vi "what_do_you_want_checkver.vi"() -> (0 "Next state":T1(ring)=enum."end", 1 "Leave":bool=TRUE)   [LabVIEW 2014]
panel:
  in  "Cluster":cluster{"OK Button 2":bool, "stop":bool}
  # "You have pressed the cancel buttom.\nWhat do you want to do now?\n1.Choose another movie.\n2.Leave the movie booking system"
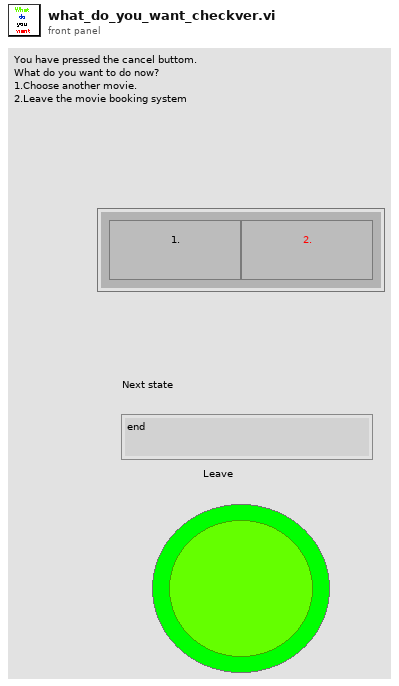
[diagram p1: front panel]
types:
  T1 = enum16{"initial", "start", "member?", "register?", "member login", "member register", "choose movie", "how many seat?", "check", "end"}
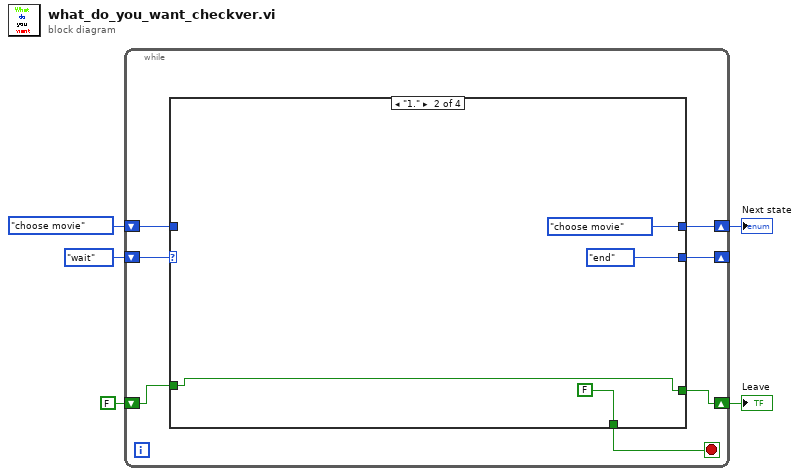
[diagram p0: block diagram]
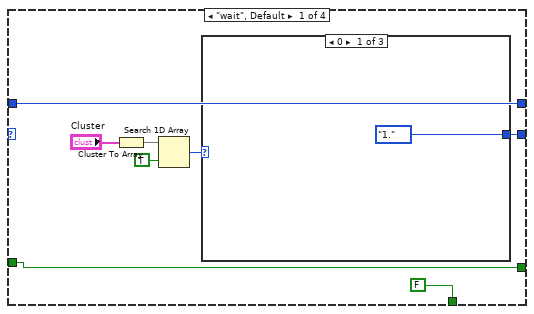
[diagram p2: hidden frame]
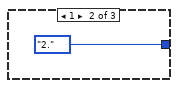
[diagram p3: hidden frame]
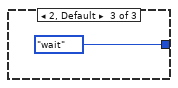
[diagram p4: hidden frame]
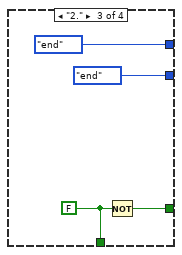
[diagram p5: hidden frame]
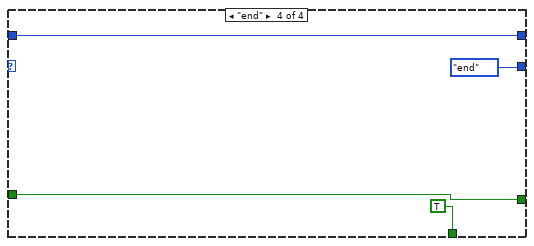
[diagram p6: hidden frame]
diagram:
  n1 = while {
    shift-right: [w11] -> _
    shift-left: enum16{"wait", "1.", "2.", "3.", "end"}."wait" -> [w12]
    shift-right: [w9] -> w3
    shift-left: T1."choose movie" -> [w10]
    shift-right: [w7] -> w1
    shift-left: FALSE -> [w6]
    stop <- w8 stop-if-true
    n2 = case shown="\"1.\"" w12 {
      tunnel: [w16 enum16{"wait", "1.", "2.", "3.", "end"}."end" enum16{"wait", "1.", "2.", "3.", "end"}."end" enum16{"wait", "1.", "2.", "3.", "end"}."end"] -> w11
      tunnel: [w15 T1."choose movie" T1."end" w34] -> w9
      tunnel: w10 -> [w15 _ _ w34]
      tunnel: [FALSE FALSE w29 TRUE] -> w8
      tunnel: [w13 w24 w28 w32] -> w7
      tunnel: w6 -> [w13 w24 _ w32]
      frame "wait", Default {
        n3 = Cluster To Array(cluster="Cluster") -> (array=w19:bool[])
        n4 = Search 1D Array(1D array=w19, element=TRUE) -> (index of element=w17:i32)  [unwired: 1 in]
        n5 = case shown="0" w17 {
          tunnel: [enum16{"wait", "1.", "2.", "3.", "end"}."1." enum16{"wait", "1.", "2.", "3.", "end"}."2." enum16{"wait", "1.", "2.", "3.", "end"}."wait"] -> w16
          frame 0 {
          }
          frame 1 {
          }
          frame 2, Default {
          }
        }
      }
      frame "1." {
      }
      frame "2." {
        w29 = FALSE
        n6 = Not(x=w29) -> (.not. x?=w28:bool)
      }
      frame "end" {
      }
    }
  }
  "Next state" <- w3
  "Leave" <- w1
